vi "Pre-Build Custom Action - EasyXML.vi"(10 "Variant":variant) -> (0 "error out":errorcluster)   [LabVIEW 2011]
uses:
  <vilib>/addons/_JKI Toolkits/VI Tester/VI Tester API.llb/Run Tests (Path).vi
  <vilib>/addons/_JKI Toolkits/VI Tester/VI Tester API.llb/VI Tester API.lvlib
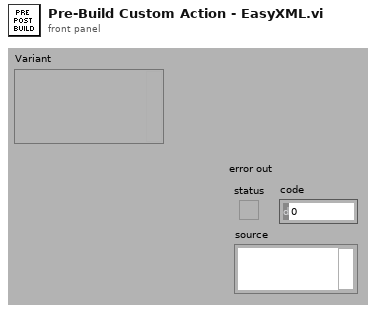
[diagram p1: front panel]
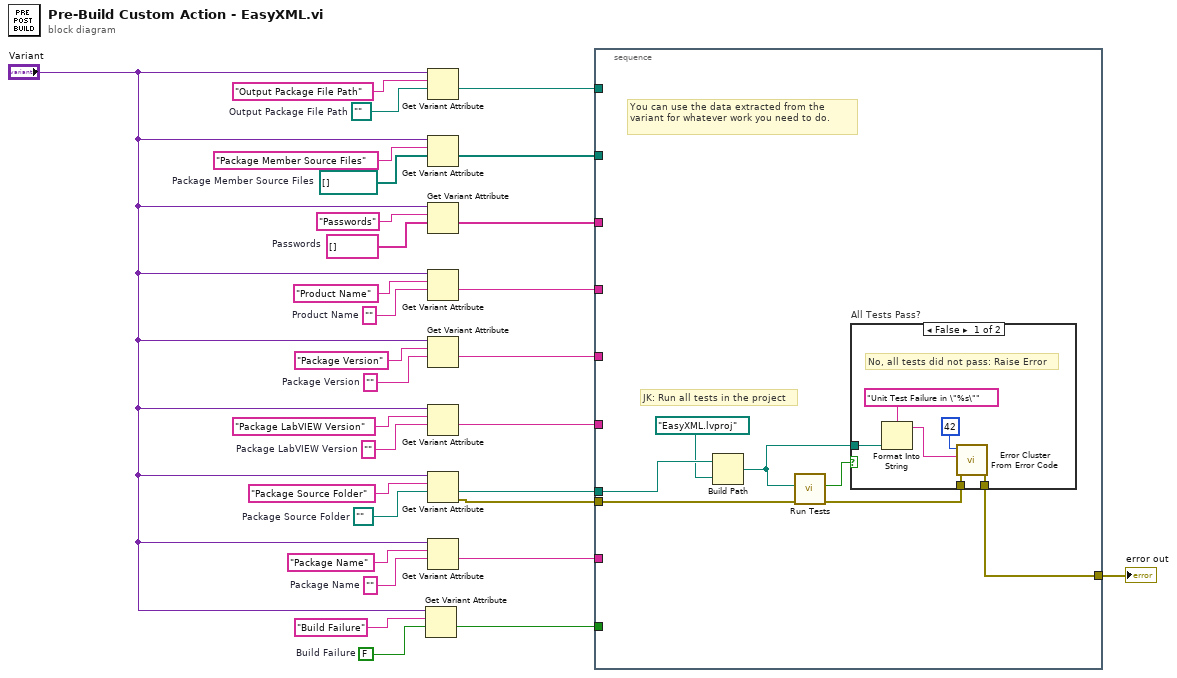
[diagram p0: block diagram]
diagram:
  w5 = FALSE  # Build Failure
  w15 = path ""  # Package Source Folder
  w16 = ""  # Package Name
  w19 = ""  # Package LabVIEW Version
  w21 = ""  # Package Version
  w23 = ""  # Product Name
  w25 = string[] []  # Passwords
  w27 = path[] []  # Package Member Source Files
  w29 = path ""  # Output Package File Path
  n1 = Get Variant Attribute(Variant="Variant", name="Build Failure", default value (empty Variant)=w5) -> (value=w3:bool)  [unwired: 1 in, 3 out]
  n2 = Get Variant Attribute(Variant="Variant", name="Output Package File Path", default value (empty Variant)=w29) -> (value=w14:path)  [unwired: 1 in, 3 out]
  n3 = Get Variant Attribute(Variant="Variant", name="Package Member Source Files", default value (empty Variant)=w27) -> (value=w13:path[])  [unwired: 1 in, 3 out]
  n4 = Get Variant Attribute(Variant="Variant", name="Passwords", default value (empty Variant)=w25) -> (value=w12:string[])  [unwired: 1 in, 3 out]
  n5 = Get Variant Attribute(Variant="Variant", name="Product Name", default value (empty Variant)=w23) -> (value=w11:string)  [unwired: 1 in, 3 out]
  n6 = Get Variant Attribute(Variant="Variant", name="Package Version", default value (empty Variant)=w21) -> (value=w10:string)  [unwired: 1 in, 3 out]
  n7 = Get Variant Attribute(Variant="Variant", name="Package LabVIEW Version", default value (empty Variant)=w19) -> (value=w9:string)  [unwired: 1 in, 3 out]
  n8 = Get Variant Attribute(Variant="Variant", name="Package Source Folder", default value (empty Variant)=w15) -> (value=w8:path, error out=w2:errorcluster)  [unwired: 1 in, 2 out]
  n9 = Get Variant Attribute(Variant="Variant", name="Package Name", default value (empty Variant)=w16) -> (value=w7:string)  [unwired: 1 in, 3 out]
  n10 = stacked-sequence {
    tunnel: w14 -> [_]
    tunnel: w13 -> [_]
    tunnel: w12 -> [_]
    tunnel: w11 -> [_]
    tunnel: w10 -> [_]
    tunnel: w9 -> [_]
    tunnel: w8 -> [w37]
    tunnel: w7 -> [_]
    tunnel: w3 -> [_]
    tunnel: w2 -> [w35]
    tunnel: [w32] -> w1
    frame #0 {
      # "JK: Run all tests in the project"
      # "You can use the data extracted from the variant for whatever work you need to do."
      n11 = Build Path(base path=w37, name or relative path=path "EasyXML.lvproj" ("base path")) -> (appended path=w31:path)
      n12 = call-poly <vilib>:"Run Tests.vi"("error in (no error)"=w35, "Test Path"=w31) -> ("error out"=w33:errorcluster, "successful?"=w34:bool)  [unwired: 7 in, 1 out]
      n13 = case "All Tests Pass?" shown="False" w34 {
        tunnel: [w42 w44] -> w32
        tunnel: w33 -> [w41 w44]
        tunnel: w31 -> [w40 _]
        frame False {
          # "No, all tests did not pass: Raise Error"
          n14 = Format Into String(format string="Unit Test Failure in \"%s\"", w40) -> (resulting string=w38:string)  [unwired: 2 in, 1 out]
          n15 = call <vilib>:"Error Cluster From Error Code.vi"("error in (no error)"=w41, "error message (\"\")"=w38, "error code (0)"=42) -> ("error out"=w42:errorcluster)  [unwired: 6 in]
        }
        frame True {
        }
      }
    }
  }
  "error out" <- w1
